vi "设备配置&联机测试.vi"(8 "error in (no error)":errorcluster caption="错误输入（无错误）") -> (0 "error out":errorcluster caption="错误输出")   [LabVIEW 2016]
uses:
  <vilib>/Utility/miscctls.llb/LVPointTypeDef.ctl
  <vilib>/ptbypt/NI_PtbyPt.lvlib
panel:
  in  "关闭":bool
  in  "联机测试":bool
  in  "选项卡控件":T1(tab)
  in  "设备列表":T2(array[cluster])
  out "波特率":u16(ring) items=["300", "600", "1200", "2400", "4800", "9600", "19200", "38400", "115200"]
  out "串口号":u16(ring) items=["COM8", "COM7", "COM6", "COM5", "COM4", "COM3", "COM2", "COM1"]
  out "就绪":bool
  in  "联机":bool
  out "航向":string
  out "速率":string
  out "经度":string
  out "纬度":string
  out "UTC时间":string
  out "UTC日期":string
  out "定位信息":string
  out "串口号 2":u16(ring) items=["COM8", "COM7", "COM6", "COM5", "COM4", "COM3", "COM2", "COM1"]
  out "就绪 2":bool
  in  "联机 2":bool caption="联机"
  in  "选项卡控件 2":T3(tab)
  in  "Turn All OFF":bool
  in  "Apply All":bool
  in  "Read Alarm Sensors":bool
  in  "Control Devices":cluster{"Name":string, "开关":bool, "状态":bool}[](array[cluster])
  in  "报警":cluster{"Name":string, " Status":bool}[](array[cluster])
  in  "Read All Sensor Values":bool
  out "T(cool)℃":string
  out "P（eq)mv":string
  out "R(Gas)mv":string
  out "F(Flow)ml/min":string
  in  "Port2":bool
  in  "Port4":bool
  in  "Port6":bool
  in  "Port8":bool
  out "串口号 4":u16(ring) items=["COM8", "COM7", "COM6", "COM5", "COM4", "COM3", "COM2", "COM1"]
  out "就绪 4":bool
  in  "联机 4":bool caption="联机"
  in  "Go":bool
  in  "Port1":bool
  in  "Port3":bool
  in  "Port5":bool
  in  "Port7":bool
  out "平均次数":dbl
  out "波特率  2":u16(ring) items=["300", "600", "1200", "2400", "4800", "9600", "19200", "38400", "115200"]
  out "串口号 3":u16(ring) items=["COM8", "COM7", "COM6", "COM5", "COM4", "COM3", "COM2", "COM1"]
  out "就绪 3":bool
  in  "联机 3":bool caption="联机"
  out "读数间隔（ms）":dbl
  out "Temperature":string
  out "Conductivity":string
  out "Salinity":string
  out "波特率":u16(ring) items=["300", "600", "1200", "2400", "4800", "9600", "19200", "38400", "115200"]
  out "串口号":u16(ring) items=["COM8", "COM7", "COM6", "COM5", "COM4", "COM3", "COM2", "COM1"]
  out "就绪 5":bool
  in  "联机 5":bool caption="联机"
  out "读数间隔 （ms）":dbl
  out "平均次数":dbl caption="数值"
  out "13CO2":string
  out "13CO2（dry）":string
  out "12CO2":string
  out "12CO2(dry）":string
  out "H2O":string
  out "Delta2Min":string
  out "Delta5Min":string
  out "波特率  3":u16(ring) items=["300", "600", "1200", "2400", "4800", "9600", "19200", "38400", "115200"]
  out "串口号":u16(ring) items=["COM8", "COM7", "COM6", "COM5", "COM4", "COM3", "COM2", "COM1"]
  out "就绪 6":bool
  in  "联机 6":bool caption="联机"
  out "读数间隔":dbl
  out "平均次数":dbl caption="数值"
  out "波特率":u16(ring) items=["300", "600", "1200", "2400", "4800", "9600", "19200", "38400", "115200"]
  out "串口号":u16(ring) items=["COM8", "COM7", "COM6", "COM5", "COM4", "COM3", "COM2", "COM1"]
  out "就绪 7":bool
  in  "联机 7":bool caption="联机"
  out "读数间隔":dbl
  out "平均次数":dbl caption="数值"
  in  "联机 8":bool caption="联机"
  out "就绪 8":bool
  out "串口号":u16(ring) items=["COM8", "COM7", "COM6", "COM5", "COM4", "COM3", "COM2", "COM1"]
  out "波特率":u16(ring) items=["300", "600", "1200", "2400", "4800", "9600", "19200", "38400", "115200"]
  out "时间":string
  out "d15NA":string
  out "d15N":string
  out "N2O":string
  out "d18O":string
  out "H2O":string
  out "d15NB":string
  out "温度摄氏度":string
  out "气压Torr":string
  out "超时us":string
  # "当前GPS信息"
  # "设置"
  # "设置"
  # "Read Temperature/Pressure sensors"
  # "逆转到1、3、5、7"
  # "设置"
  # "设置"
  # "就绪4"
  # "设置"
  # "DATA"
  # "设置"
  # "设置"
  # "设置"
  # "DATA"
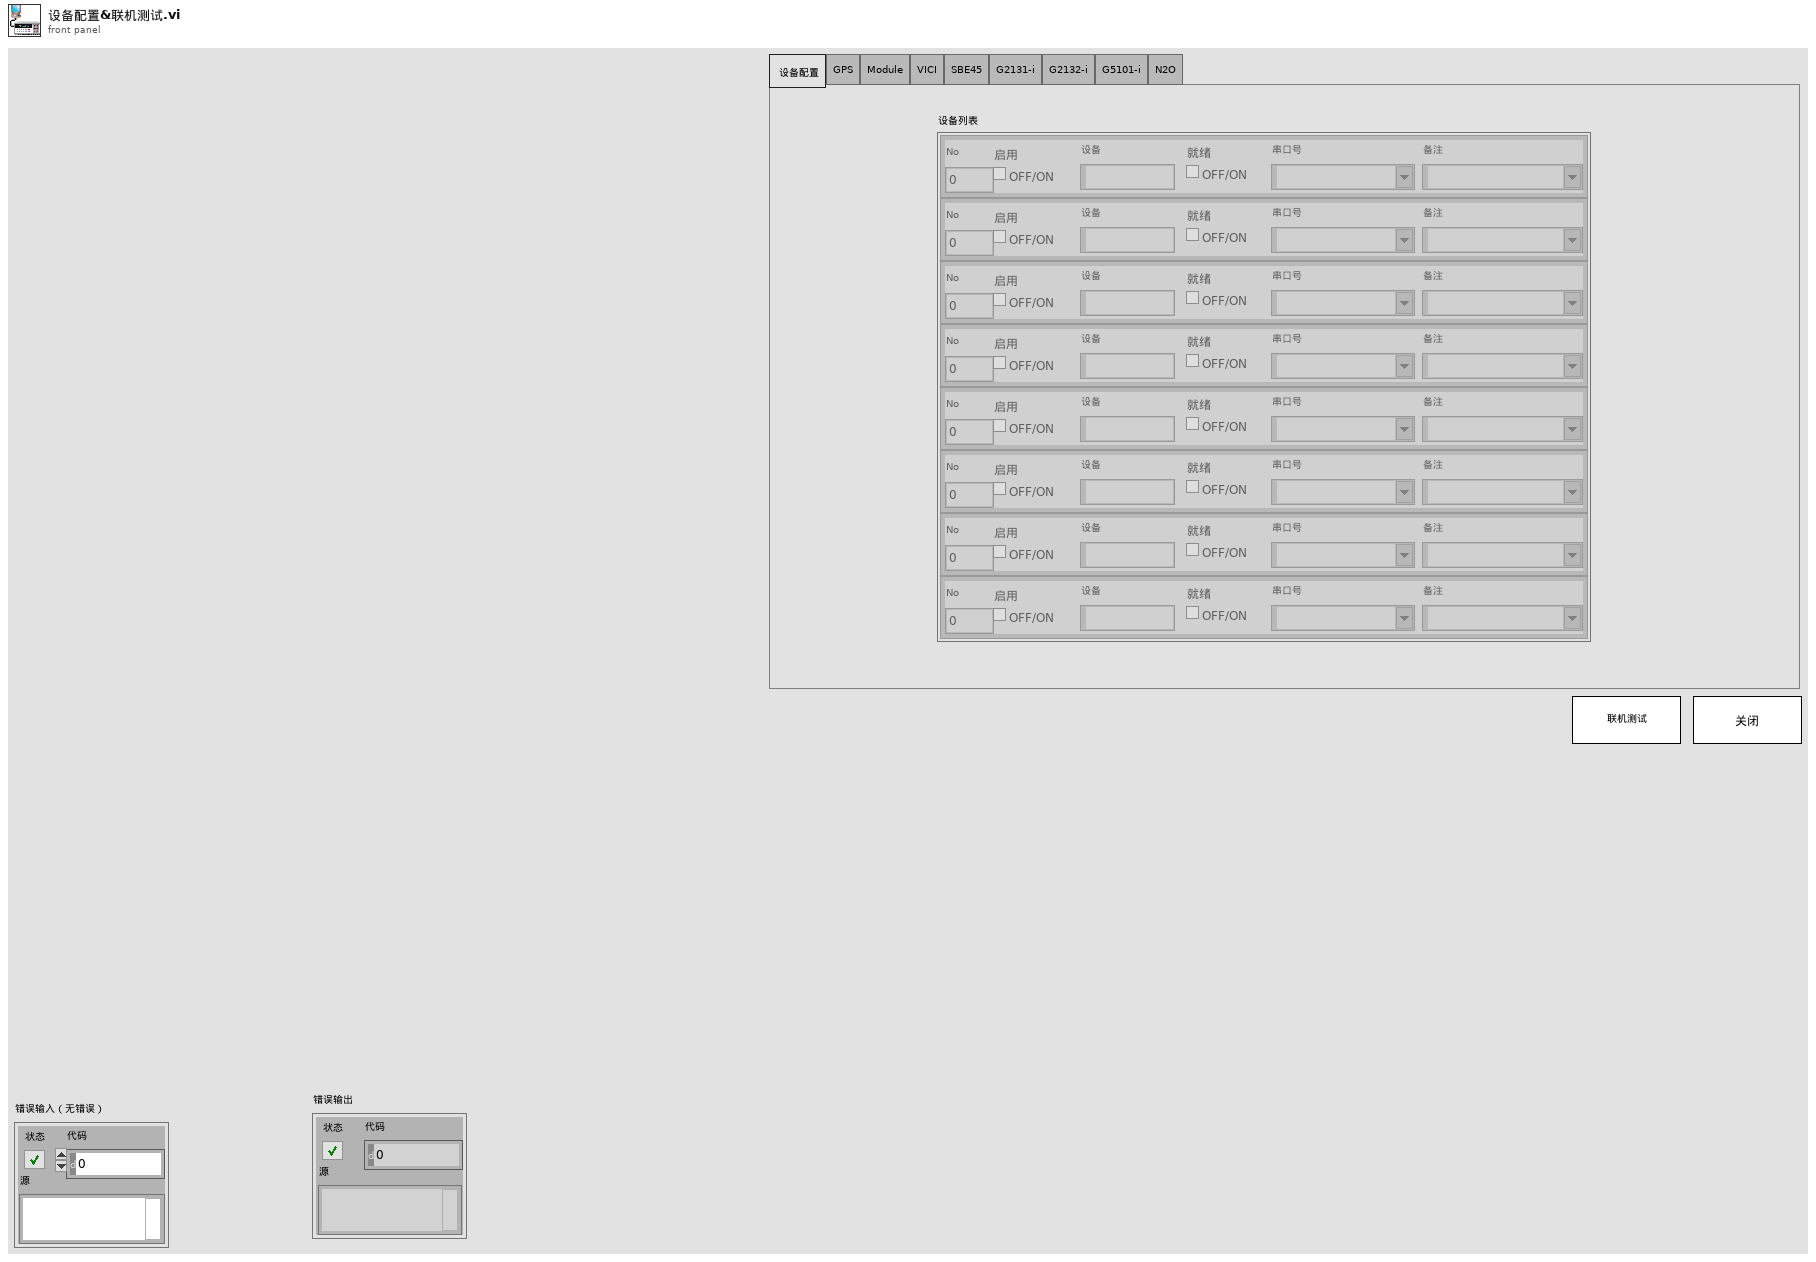
[diagram p1: front panel]
types:
  T1 = enum32{" 设备配置", "GPS", "Module", "VICI", "SBE45", "G2131-i", "G2132-i", "G5101-i", "N2O"}
  T2 = cluster{"No":dbl, "启用":bool, "设备":string, "就绪 ":bool, "串口号":string, "备注":string}[]
  T3 = enum32{"Control Devices&Other Sensors", "T|P|R|F Sensors"}
  T4 = typedef "LVPointTypeDef.ctl" = cluster{"Horizontal":i16, "Vertical":i16}
  T5 = cluster{"No":dbl, "启用":bool, "设备":string, "就绪 ":bool, "串口号":string, "备注":string}
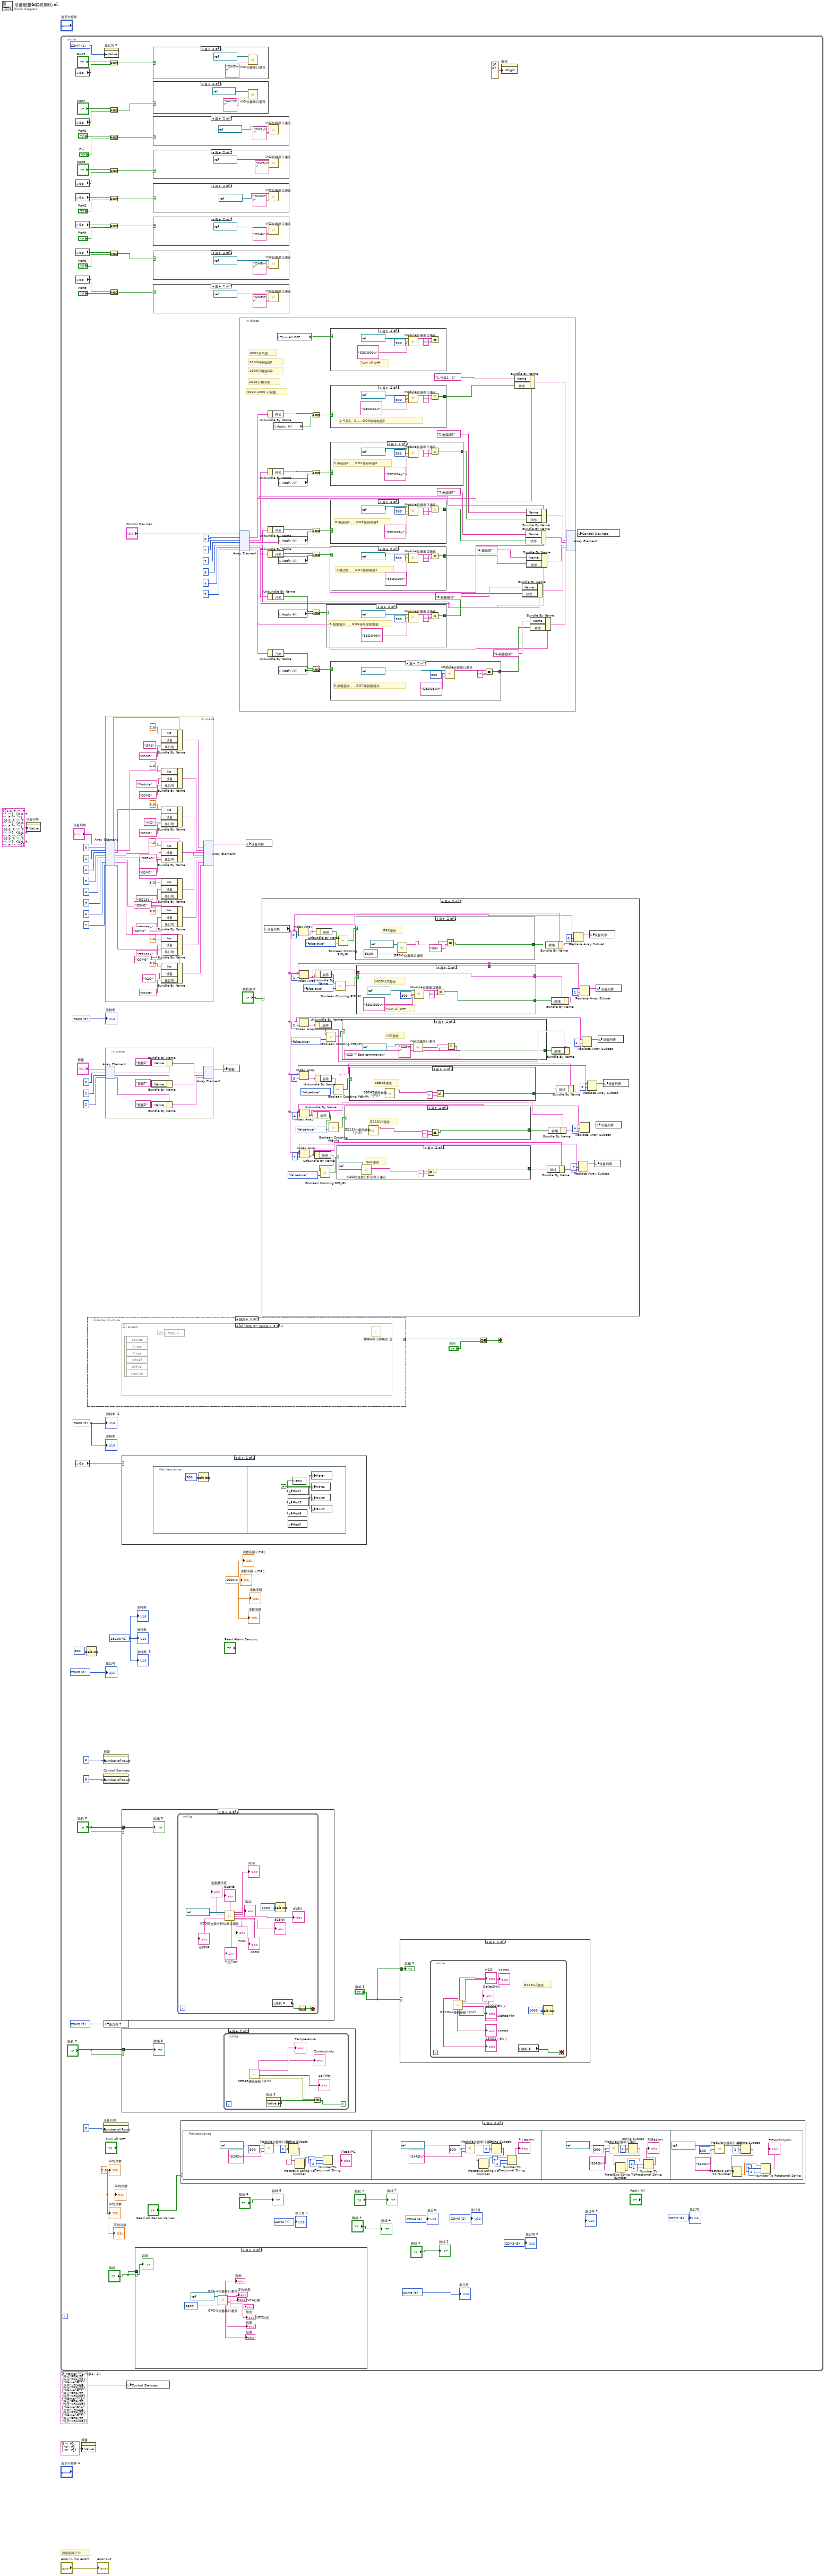
[diagram p0: block diagram]
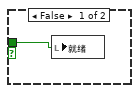
[diagram p9: hidden frame]
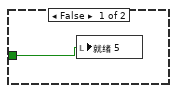
[diagram p10: hidden frame]
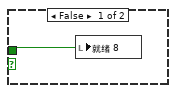
[diagram p11: hidden frame]
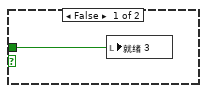
[diagram p17: hidden frame]
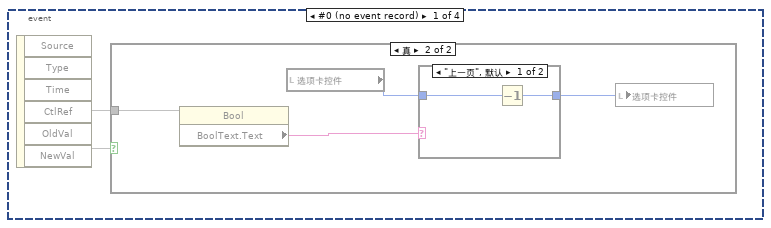
[diagram p18: hidden frame]
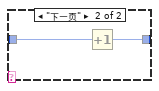
[diagram p20: hidden frame]
diagram:
  # "调用各种子VI"
  n1 = property on="设备列表" class="Arr (严格)"("Value"=T2 [{"No"=1.0, "启用"=FALSE, "设备"="", "就绪 "=FALSE, "串口号"="", "备注"=""}, {"No"=0.0, "启用"=FALSE, "设备"="", "就绪 "=FALSE, "串口号"="", "备注"=""}, {"No"=0.0, "启用"=FALSE, "设备"="", "就绪 "=FALSE, "串口号"="", "备注"=""}, {"No"=0.0, "启用"=FALSE, "设备"="", "就绪 "=FALSE, "串口号"="", "备注"=""}, {"No"=0.0, "启用"=FALSE, "设备"="", "就绪 "=FALSE, "串口号"="", "备注"=""}, {"No"=0.0, "启用"=FALSE, "设备"="", "就绪 "=FALSE, "串口号"="", "备注"=""}, {"No"=0.0, "启用"=FALSE, "设备"="", "就绪 "=FALSE, "串口号"="", "备注"=""}, {"No"=0.0, "启用"=FALSE, "设备"="", "就绪 "=FALSE, "串口号"="", "备注"=""}] ("设备列表")) -> ()  [unwired: 2 in, 2 out]
  n2 = while {
    stop <- w48 stop-if-true
    w12 = u16 5 items=["COM8", "COM7", "COM6", "COM5", "COM4", "COM3", "COM2", "COM1"] ("串口号 2")
    w14 = 1.0 ("平均次数")
    w13 = 1000.0 ("读数间隔 2")
    w18 = u16 2 items=["COM8", "COM7", "COM6", "COM5", "COM4", "COM3", "COM2", "COM1"] ("串口号 7")
    w19 = u16 4 items=["COM8", "COM7", "COM6", "COM5", "COM4", "COM3", "COM2", "COM1"] ("串口号 6")
    w20 = u16 6 items=["COM8", "COM7", "COM6", "COM5", "COM4", "COM3", "COM2", "COM1"] ("串口号 5")
    w21 = u16 7 items=["COM8", "COM7", "COM6", "COM5", "COM4", "COM3", "COM2", "COM1"] ("串口号 4")
    w23 = u16 5 items=["300", "600", "1200", "2400", "4800", "9600", "19200", "38400", "115200"] ("波特率  5")
    w24 = u16 0 items=["COM8", "COM7", "COM6", "COM5", "COM4", "COM3", "COM2", "COM1"] ("串口号 8")
    w26 = u16 5 items=["300", "600", "1200", "2400", "4800", "9600", "19200", "38400", "115200"] ("波特率")
    w27 = u16 6 items=["300", "600", "1200", "2400", "4800", "9600", "19200", "38400", "115200"] ("波特率  4")
    w15 = u16 3 items=["COM8", "COM7", "COM6", "COM5", "COM4", "COM3", "COM2", "COM1"] ("串口号")
    w42 = u16 5 items=["COM8", "COM7", "COM6", "COM5", "COM4", "COM3", "COM2", "COM1"] ("串口号 2")
    w43 = u16 1 items=["COM8", "COM7", "COM6", "COM5", "COM4", "COM3", "COM2", "COM1"] ("串口号 3")
    n3 = local read "Go"() -> (w52:bool)
    n4 = local read "Go"() -> (w51:bool)
    n5 = local read "Go"() -> (w53:bool)
    n6 = local read "Go"() -> (w41:bool)
    n7 = local read "Go"() -> (w38:bool)
    n8 = local read "Go"() -> (w35:bool)
    n9 = local read "Go"() -> (w32:bool)
    n10 = local read "Go"() -> (w29:bool)
    n11 = Wait (ms)(milliseconds to wait=u32 300 ("等待时间（毫秒）")) -> ()  [unwired: 1 out]
    n12 = disable-structure shown="禁用" {
      disable-tunnel: [w226 _] -> w49
      frame Disabled {
        n13 = event shown="[2] \"联机 2\": 值改变" {
          selector: _ -> [_ _ _ _]
          dyn-events: _ -> [_ _ _ _]
          timeout: _ -> [_ _ _ _]
          tunnel: [_ _ _ TRUE] -> w226
          event #0 (no event record) {
            n14 = event-data() -> ("CtlRef"=w228, "NewVal"=w227)  [unwired: 1 in, 4 out]
            n15 = case shown="真" w227 {
              tunnel: w228 -> [_ w232]
              frame False {
              }
              frame True {
                n16 = property class="Bool"(reference=w232) -> ("BoolText.Text"=w231:string)  [unwired: 1 in, 2 out]
                n17 = local read "选项卡控件"() -> (w230:T1)
                n18 = case shown="\"上一页\", 默认" w231 {
                  tunnel: w230 -> [w234 w236]
                  tunnel: [w233 w235] -> w229
                  frame "上一页", Default {
                    n19 = Decrement(x=w234) -> (x-1=w233:T1)
                  }
                  frame "下一页" {
                    n20 = Increment(x=w236) -> (x+1=w235:T1)
                  }
                }
                n21 = local write "选项卡控件"(w229) -> ()
              }
            }
          }
          event #1 (no event record) {
            n22 = event-data() -> ("CtlRef"=w238, "OldVal"=w237)  [unwired: 1 in, 4 out]
            n23 = case shown="真" w237 {
              tunnel: w238 -> [_ w242]
              frame False {
              }
              frame True {
                n24 = property class="Bool (严格)"(reference=w242) -> ("BoolText.Text"=w241:string)  [unwired: 1 in, 2 out]
                n25 = local read "选项卡控件"() -> (w240:T1)
                n26 = case shown="\"下一页\", 默认" w241 {
                  tunnel: w240 -> [w244 w246]
                  tunnel: [w243 w245] -> w239
                  frame "下一页", Default {
                    n27 = Increment(x=w244) -> (x+1=w243:T1)
                  }
                  frame "上一页" {
                    n28 = Decrement(x=w246) -> (x-1=w245:T1)
                  }
                }
                n29 = local write "选项卡控件"(w239) -> ()
              }
            }
          }
          event "联机 2": Value Change {
            n30 = event-data() -> ()  [unwired: 1 in, 6 out]
            n31 = local write "联机 2"(FALSE) -> ()
            n32 = call "模块1串口初始化.vi"() -> ()  [unwired: 12 in]
          }
          event "关闭": Value Change {
            n33 = event-data() -> ()  [unwired: 1 in, 6 out]
          }
        }
      }
      frame Enabled {
      }
    }
    n34 = property on="报警" class="Arr (严格)"("Number of Rows"=u32 3 ("行数")) -> ()  [unwired: 2 in, 2 out]
    n35 = property on="Control Devices" class="Arr (严格)"("Number of Rows"=u32 6 ("行数")) -> ()  [unwired: 2 in, 2 out]
    n36 = property on="设备列表" class="Arr (严格)"("Number of Rows"=u32 8 ("行数")) -> ()  [unwired: 2 in, 2 out]
    n37 = local write "串口号 2"(w42) -> ()
    n38 = property on="串口号 3" class="Ring (严格)"("Value"=w43) -> ()  [unwired: 2 in, 2 out]
    n39 = in-place {
      n40 = in-place-array #1("设备列表", 0, 1, 2 ("数值"), 3, 4, 5, 6, 7) -> (w424:T5, w423:T5, w422:T5, w416:T5, w410:T5, w409:T5, w405:T5, w398:T5)
      n41 = Bundle By Name(cluster=w424, "No"=1.0 ("数值"), "设备"="GPS" ("字符串"), "串口号"="COM5") -> (w430:T5)
      n42 = Bundle By Name(cluster=w423, "No"=2.0, "设备"="Module", "串口号"="COM3") -> (w425:T5)
      n43 = Bundle By Name(cluster=w422, "No"=3.0, "设备"="VICI", "串口号"="COM1") -> (w421:T5)
      n44 = Bundle By Name(cluster=w416, "No"=4.0, "设备"="SBE45", "串口号"="COM7") -> (w415:T5)
      n45 = Bundle By Name(cluster=w410, "No"=5.0, "设备"="G2131-i", "串口号"="COM2") -> (w408:T5)
      n46 = Bundle By Name(cluster=w409, "No"=6.0, "设备"="G2132-i", "串口号"="COM4") -> (w407:T5)
      n47 = Bundle By Name(cluster=w405, "No"=7.0, "设备"="G5101-i", "串口号"="COM6") -> (w404:T5)
      n48 = Bundle By Name(cluster=w398, "No"=8.0, "设备"="N2O", "串口号"="COM8") -> (w397:T5)
      n49 = in-place-array #1(w430, w425, w421, w415, w408, w407, w404, w397) -> (w77:T2)  [unwired: 8 out]
    }
    n50 = in-place {
      n51 = in-place-array #2("报警", 0, 1, 2) -> (w305:cluster{"Name":string, " Status":bool}, w302:cluster{"Name":string, " Status":bool}, w299:cluster{"Name":string, " Status":bool})
      n52 = Bundle By Name(cluster=w305, "Name"="报警1") -> (w304:cluster{"Name":string, " Status":bool})
      n53 = Bundle By Name(cluster=w302, "Name"="报警2") -> (w301:cluster{"Name":string, " Status":bool})
      n54 = Bundle By Name(cluster=w299, "Name"="报警3") -> (w300:cluster{"Name":string, " Status":bool})
      n55 = in-place-array #2(w304, w301, w300) -> (w62:cluster{"Name":string, " Status":bool}[])  [unwired: 3 out]
    }
    n56 = And(x="Port5", y=w52) -> (x .and. y?=w55:bool)
    n57 = And(x="Port7", y=w51) -> (x .and. y?=w54:bool)
    n58 = And(x="Port1", y="Go") -> (x .and. y?=w57:bool)
    n59 = And(x="Port3", y=w53) -> (x .and. y?=w56:bool)
    n60 = And(x=w41, y="Port2") -> (x .and. y?=w39:bool)
    n61 = And(x=w38, y="Port4") -> (x .and. y?=w36:bool)
    n62 = And(x=w35, y="Port6") -> (x .and. y?=w33:bool)
    n63 = And(x=w32, y="Port8") -> (x .and. y?=w30:bool)
    n64 = case shown="真" w29 {
      frame False {
      }
      frame True {
        n65 = flat-sequence {
          frame #0 {
            n66 = Wait (ms)(milliseconds to wait=u32 500 ("等待时间（毫秒）")) -> ()  [unwired: 1 out]
          }
          frame #1 {
            w209 = FALSE
            n67 = local write "Port1"(w209) -> ()
            n68 = local write "Port3"(w209) -> ()
            n69 = local write "Port5"(w209) -> ()
            n70 = local write "Port7"(w209) -> ()
            n71 = local write "Go"(w209) -> ()
            n72 = local write "Port4"(w209) -> ()
            n73 = local write "Port6"(w209) -> ()
            n74 = local write "Port8"(w209) -> ()
            n75 = local write "Port2"(w209) -> ()
          }
        }
      }
    }
    n76 = case shown="真" "联机 8" {
      tunnel: "联机 8" -> [w192 w193]
      frame False {
        n77 = local write "就绪 8"(w192) -> ()
      }
      frame True {
        n78 = while {
          stop <- w203 stop-if-true
          n79 = call "N2O同位素分析仪串口通讯.vi"("VISA resource name"=refnum<visa-resource-name> "COM8") -> ("温度摄氏度"=→"温度摄氏度":string, "d15NB"=→"d15NB":string, "时间"=→"时间":string, "N2O"=→"N2O":string, "d15N"=→"d15N":string, "d18O"=→"d18O":string, "超时us"=→"超时us":string, "气压Torr"=→"气压Torr":string, "H2O"=→"H2O":string, "d15NA"=→"d15NA":string)  [unwired: 5 in]
          n80 = local read "联机 8"() -> (w204:bool)
          n81 = Wait (ms)(milliseconds to wait=u32 1000 ("等待时间（毫秒）")) -> ()  [unwired: 1 out]
          n82 = Not(x=w204) -> (.not. x?=w203:bool)
        }
        "就绪 8" <- w193
      }
    }
    n83 = case shown="真" "联机 3" {
      tunnel: "联机 3" -> [w218 w219]
      frame False {
        n84 = local write "就绪 3"(w218) -> ()
      }
      frame True {
        n85 = while {
          stop <- w221 continue-if-true
          n86 = call "SBE45通讯参数 (子VI).vi"() -> ("错误输出"=w222:errorcluster, "Salinity"=→"Salinity":string, "Conductivity"=→"Conductivity":string, "Temperature"=→"Temperature":string)  [unwired: 8 in]
          n87 = property on="联机 3" class="Bool (严格)"() -> ("Value"=w220:bool)  [unwired: 2 in, 2 out]
          n88 = Or(x=w222, y=w220) -> (x .or. y?=w221:bool)
        }
        "就绪 3" <- w219
      }
    }
    n89 = case shown="真" "联机" {
      selector: "联机" -> [_ w178]
      tunnel: "联机" -> [w168 _]
      frame False {
        n90 = local write "就绪"(w168) -> ()
      }
      frame True {
        n91 = call "GPS-1仪器串口通讯.vi"("VISA resource name"=refnum<visa-resource-name> "COM5", "baud rate (9600)"=u32 9600) -> ()  [unwired: 10 in, 8 out]
        n92 = call "GPS-1仪器串口通讯.vi"("VISA resource name"=refnum<visa-resource-name> "COM5", "baud rate (9600)"=u32 9600) -> ("速率"=→"速率":string, "经度"=→"经度":string, "定位信息"=→"定位信息":string, "UTC日期"=→"UTC日期":string, "航向"=→"航向":string, "UTC时间"=→"UTC时间":string, "纬度"=→"纬度":string)  [unwired: 10 in, 1 out]
        "就绪" <- w178
      }
    }
    n93 = case shown="真" w55 {
      frame False {
      }
      frame True {
        n94 = call "VICI仪器串口通讯.vi"("输入指令"="CW5\n\r", "VISA resource name"=refnum<visa-resource-name> "COM1") -> ()  [unwired: 1 in, 3 out]
      }
    }
    n95 = case shown="真" w54 {
      frame False {
      }
      frame True {
        n96 = call "VICI仪器串口通讯.vi"("输入指令"="CW7\n\r", "VISA resource name"=refnum<visa-resource-name> "COM1") -> ()  [unwired: 1 in, 3 out]
      }
    }
    n97 = case shown="真" w57 {
      frame False {
      }
      frame True {
        n98 = call "VICI仪器串口通讯.vi"("输入指令"="CW1\n\r", "VISA resource name"=refnum<visa-resource-name> "COM1") -> ()  [unwired: 1 in, 3 out]
      }
    }
    n99 = case shown="真" w56 {
      frame False {
      }
      frame True {
        n100 = call "VICI仪器串口通讯.vi"("输入指令"="CW3\n\r", "VISA resource name"=refnum<visa-resource-name> "COM1") -> ()  [unwired: 1 in, 3 out]
      }
    }
    n101 = case shown="真" w39 {
      frame False {
      }
      frame True {
        n102 = call "VICI仪器串口通讯.vi"("输入指令"="CW2\n\r", "VISA resource name"=refnum<visa-resource-name> "COM1") -> ()  [unwired: 1 in, 3 out]
      }
    }
    n103 = case shown="真" w36 {
      frame False {
      }
      frame True {
        n104 = call "VICI仪器串口通讯.vi"("输入指令"="CW4\r", "VISA resource name"=refnum<visa-resource-name> "COM1") -> ()  [unwired: 1 in, 3 out]
      }
    }
    n105 = case shown="真" w33 {
      frame False {
      }
      frame True {
        n106 = call "VICI仪器串口通讯.vi"("输入指令"="CW6\n\r", "VISA resource name"=refnum<visa-resource-name> "COM1") -> ()  [unwired: 1 in, 3 out]
      }
    }
    n107 = case shown="真" w30 {
      frame False {
      }
      frame True {
        n108 = call "VICI仪器串口通讯.vi"("输入指令"="CW8\n\r", "VISA resource name"=refnum<visa-resource-name> "COM1") -> ()  [unwired: 1 in, 3 out]
      }
    }
    n109 = case shown="真" "Read All Sensor Values" {
      frame False {
      }
      frame True {
        n110 = flat-sequence {
          frame #0 {
            n111 = call "Module仪器串口通讯.vi"("输入指令"="$2RD\r", "baud rate"=u32 300 ("baud rate (9600)"), "VISA resource name"=refnum<visa-resource-name> "COM3") -> ("子字符串;substring"=w254:string)  [unwired: 2 out]
            n112 = String Subset(string=w254, offset (0)=2 ("偏移量(0)")) -> (substring=w253:string)  [unwired: 1 in]
            n113 = Fract/Exp String To Number(string=w253) -> (number=w252:dbl)  [unwired: 3 in, 1 out]
            n114 = Number To Fractional String(number=w252, width (-)=i16 2 ("宽度(-)"), precision (6)=i16 2 ("精度(6)")) -> (F-format string=→"T(cool)℃":string)  [unwired: 1 in]
          }
          frame #1 {
            n115 = call "Module仪器串口通讯.vi"("输入指令"="$4RD\r", "baud rate"=u32 300 ("baud rate (9600)"), "VISA resource name"=refnum<visa-resource-name> "COM3") -> ("子字符串;substring"=w264:string)  [unwired: 2 out]
            n116 = String Subset(string=w264, offset (0)=2 ("偏移量(0)")) -> (substring=w260:string)  [unwired: 1 in]
            n117 = Fract/Exp String To Number(string=w260) -> (number=w263:dbl)  [unwired: 3 in, 1 out]
            n118 = Number To Fractional String(number=w263, width (-)=i16 2 ("宽度(-)"), precision (6)=i16 2 ("精度(6)")) -> (F-format string=→"P（eq)mv":string)  [unwired: 1 in]
          }
          frame #2 {
            n119 = call "Module仪器串口通讯.vi"("输入指令"="$5RD\r", "baud rate"=u32 300 ("baud rate (9600)"), "VISA resource name"=refnum<visa-resource-name> "COM3") -> ("子字符串;substring"=w274:string)  [unwired: 2 out]
            n120 = String Subset(string=w274, offset (0)=2 ("偏移量(0)")) -> (substring=w270:string)  [unwired: 1 in]
            n121 = Fract/Exp String To Number(string=w270) -> (number=w271:dbl)  [unwired: 3 in, 1 out]
            n122 = Number To Fractional String(number=w271, width (-)=i16 2 ("宽度(-)"), precision (6)=i16 2 ("精度(6)")) -> (F-format string=→"R(Gas)mv":string)  [unwired: 1 in]
          }
          frame #3 {
            n123 = call "Module仪器串口通讯.vi"("输入指令"="$6RD\r", "baud rate"=u32 300 ("baud rate (9600)"), "VISA resource name"=refnum<visa-resource-name> "COM3") -> ("子字符串;substring"=w288:string)  [unwired: 2 out]
            n124 = String Subset(string=w288, offset (0)=2 ("偏移量(0)")) -> (substring=w280:string)  [unwired: 1 in]
            n125 = Fract/Exp String To Number(string=w280) -> (number=w283:dbl)  [unwired: 3 in, 1 out]
            n126 = Number To Fractional String(number=w283, width (-)=i16 2 ("宽度(-)"), precision (6)=i16 2 ("精度(6)")) -> (F-format string=→"F(Flow)ml/min":string)  [unwired: 1 in]
          }
        }
      }
    }
    n127 = local write "报警"(w62) -> ()
    n128 = in-place {
      # "0010 1000 开报警"
      # "1010开蠕动泵"
      # "1000开电磁阀2"
      # "0100开电磁阀1"
      # "0001开气泵"
      n129 = in-place-array #3("Control Devices", 0, 1, 2, 3, 4, 5) -> (w319:cluster{"Name":string, "开关":bool, "状态":bool}, w320:cluster{"Name":string, "开关":bool, "状态":bool}, w321:cluster{"Name":string, "开关":bool, "状态":bool}, w327:cluster{"Name":string, "开关":bool, "状态":bool}, w332:cluster{"Name":string, "开关":bool, "状态":bool}, w331:cluster{"Name":string, "开关":bool, "状态":bool})
      n130 = Unbundle By Name(w319) -> ("开关"=w322:bool)
      n131 = Unbundle By Name(w320) -> ("开关"=w323:bool)
      n132 = Unbundle By Name(w321) -> ("开关"=w326:bool)
      n133 = Unbundle By Name(w327) -> ("开关"=w330:bool)
      n134 = Unbundle By Name(w332) -> ("开关"=w336:bool)
      n135 = Unbundle By Name(w331) -> ("开关"=w333:bool)
      n136 = local read "Apply All"() -> (w306:bool)
      n137 = local read "Turn All OFF"() -> (w318:bool)
      n138 = local read "Apply All"() -> (w324:bool)
      n139 = local read "Apply All"() -> (w325:bool)
      n140 = local read "Apply All"() -> (w329:bool)
      n141 = local read "Apply All"() -> (w335:bool)
      n142 = local read "Apply All"() -> (w310:bool)
      n143 = And(x=w322, y=w306) -> (x .and. y?=w307:bool)
      n144 = And(x=w323, y=w324) -> (x .and. y?=w308:bool)
      n145 = And(x=w326, y=w325) -> (x .and. y?=w309:bool)
      n146 = And(x=w330, y=w329) -> (x .and. y?=w328:bool)
      n147 = And(x=w336, y=w335) -> (x .and. y?=w334:bool)
      n148 = And(x=w333, y=w310) -> (x .and. y?=w317:bool)
      n149 = case shown="真" w334 {
        tunnel: [_ w385] -> w314
        frame False {
        }
        frame True {
          # "5.报警器开，，DO6接外部报警器"
          n150 = call "Module仪器串口通讯.vi"("输入指令"="$3DO40\r", "baud rate"=u32 300 ("baud rate (9600)"), "VISA resource name"=refnum<visa-resource-name> "COM3") -> ("子字符串;substring"=w386:string)  [unwired: 2 out]
          n151 = Equal?(x=w386, y="*") -> (x = y?=w385:bool)
        }
      }
      n152 = case shown="真" w318 {
        frame False {
        }
        frame True {
          # "Turn All OFF"
          n153 = call "Module仪器串口通讯.vi"("输入指令"="$3DO00\r", "baud rate"=u32 300 ("baud rate (9600)"), "VISA resource name"=refnum<visa-resource-name> "COM3") -> ("子字符串;substring"=w349:string)  [unwired: 2 out]
          n154 = Equal?(x=w349, y="*") -> ()  [unwired: 1 out]
        }
      }
      n155 = case shown="真" w307 {
        tunnel: [_ w354] -> w316
        frame False {
        }
        frame True {
          # "1.气泵1、2,,,,,,DO0接继电器0"
          n156 = call "Module仪器串口通讯.vi"("输入指令"="$3DO01\r", "baud rate"=u32 300 ("baud rate (9600)"), "VISA resource name"=refnum<visa-resource-name> "COM3") -> ("子字符串;substring"=w355:string)  [unwired: 2 out]
          n157 = Equal?(x=w355, y="*") -> (x = y?=w354:bool)
        }
      }
      n158 = case shown="真" w308 {
        tunnel: [FALSE w361] -> w311
        frame False {
        }
        frame True {
          # "2.电磁阀1，，DO2接继电器2"
          n159 = call "Module仪器串口通讯.vi"("输入指令"="$3DO04\r", "baud rate"=u32 300 ("baud rate (9600)"), "VISA resource name"=refnum<visa-resource-name> "COM3") -> ("子字符串;substring"=w362:string)  [unwired: 2 out]
          n160 = Equal?(x=w362, y="*") -> (x = y?=w361:bool)
        }
      }
      n161 = case shown="真" w309 {
        tunnel: [_ w367] -> w312
        frame False {
        }
        frame True {
          # "3.电磁阀2，，DO3接继电器3"
          n162 = call "Module仪器串口通讯.vi"("输入指令"="$3DO08\r", "baud rate"=u32 300 ("baud rate (9600)"), "VISA resource name"=refnum<visa-resource-name> "COM3") -> ("子字符串;substring"=w368:string)  [unwired: 2 out]
          n163 = Equal?(x=w368, y="*") -> (x = y?=w367:bool)
        }
      }
      n164 = case shown="真" w328 {
        tunnel: [_ w373] -> w313
        frame False {
        }
        frame True {
          # "4.蠕动泵，，DO4接继电器4"
          n165 = call "Module仪器串口通讯.vi"("输入指令"="$3DO10\r", "baud rate"=u32 300 ("baud rate (9600)"), "VISA resource name"=refnum<visa-resource-name> "COM3") -> ("子字符串;substring"=w374:string)  [unwired: 2 out]
          n166 = Equal?(x=w374, y="*") -> (x = y?=w373:bool)
        }
      }
      n167 = case shown="真" w317 {
        tunnel: [_ w379] -> w315
        frame False {
        }
        frame True {
          # "6.报警器关，，DO7接报警器关"
          n168 = call "Module仪器串口通讯.vi"("输入指令"="$3DO80\r", "baud rate"=u32 300 ("baud rate (9600)"), "VISA resource name"=refnum<visa-resource-name> "COM3") -> ("子字符串;substring"=w380:string)  [unwired: 2 out]
          n169 = Equal?(x=w380, y="*") -> (x = y?=w379:bool)
        }
      }
      n170 = Bundle By Name(cluster=w319, "Name"="1.气泵1、2" ("字符串"), "状态"=w316) -> (w348:cluster{"Name":string, "开关":bool, "状态":bool})
      n171 = Bundle By Name(cluster=w332, "Name"="5.报警器开" ("字符串"), "状态"=w314) -> (w338:cluster{"Name":string, "开关":bool, "状态":bool})
      n172 = Bundle By Name(cluster=w321, "Name"="3.电磁阀2" ("字符串"), "状态"=w312) -> (w340:cluster{"Name":string, "开关":bool, "状态":bool})
      n173 = Bundle By Name(cluster=w320, "Name"="2.电磁阀1" ("字符串"), "状态"=w311) -> (w341:cluster{"Name":string, "开关":bool, "状态":bool})
      n174 = Bundle By Name(cluster=w327, "Name"="4.蠕动泵" ("字符串"), "状态"=w313) -> (w339:cluster{"Name":string, "开关":bool, "状态":bool})
      n175 = Bundle By Name(cluster=w331, "Name"="6.报警器关" ("字符串"), "状态"=w315) -> (w337:cluster{"Name":string, "开关":bool, "状态":bool})
      n176 = in-place-array #3(w348, w341, w340, w339, w338, w337) -> (w72:cluster{"Name":string, "开关":bool, "状态":bool}[])  [unwired: 6 out]
    }
    n177 = local write "设备列表"(w77) -> ()
    n178 = case shown="真" "联机测试" {
      frame False {
      }
      frame True {
        n179 = local read "设备列表"() -> (w106:T2)
        n180 = Index Array(array=w106, index=0 ("索引")) -> (element=w125:T5)
        n181 = Index Array(array=w106, index=2 ("索引")) -> (element=w120:T5)
        n182 = Index Array(array=w106, index=3 ("索引")) -> (element=w117:T5)
        n183 = Index Array(array=w106, index=1 ("索引")) -> (element=w139:T5)
        n184 = Index Array(array=w106, index=4 ("索引")) -> (element=w110:T5)
        n185 = Index Array(array=w106, index=7 ("索引")) -> (element=w107:T5)
        n186 = Unbundle By Name(w110) -> ("启用"=w85:bool)
        n187 = Unbundle By Name(w107) -> ("启用"=w87:bool)
        n188 = Unbundle By Name(w120) -> ("启用"=w94:bool)
        n189 = Unbundle By Name(w139) -> ("启用"=w102:bool)
        n190 = Unbundle By Name(w117) -> ("启用"=w91:bool)
        n191 = Unbundle By Name(w125) -> ("启用"=w98:bool)
        n192 = call <vilib>:"Boolean Crossing PtByPt.vi"("direction"=enum16{"either", "false-true", "true-false"}."false-true", "input"=w87) -> ("crossing"=w88:bool)  [unwired: 1 in]
        n193 = call <vilib>:"Boolean Crossing PtByPt.vi"("direction"=enum16{"either", "false-true", "true-false"}."false-true", "input"=w94) -> ("crossing"=w95:bool)  [unwired: 1 in]
        n194 = call <vilib>:"Boolean Crossing PtByPt.vi"("direction"=enum16{"either", "false-true", "true-false"}."false-true", "input"=w85) -> ("crossing"=w86:bool)  [unwired: 1 in]
        n195 = call <vilib>:"Boolean Crossing PtByPt.vi"("direction"=enum16{"either", "false-true", "true-false"}."false-true", "input"=w91) -> ("crossing"=w92:bool)  [unwired: 1 in]
        n196 = call <vilib>:"Boolean Crossing PtByPt.vi"("direction"=enum16{"either", "false-true", "true-false"}."false-true", "input"=w102) -> ("crossing"=w101:bool)  [unwired: 1 in]
        n197 = case shown="真" w88 {
          tunnel: [_ w141] -> w105
          frame False {
          }
          frame True {
            # "N2O通信"
            n198 = call "N2O同位素分析仪串口通讯.vi"("VISA resource name"=refnum<visa-resource-name> "COM8") -> ("时间"=w143:string)  [unwired: 5 in, 9 out]
            n199 = Not Equal?(x=w143, y="") -> (x != y?=w141:bool)
          }
        }
        n200 = call <vilib>:"Boolean Crossing PtByPt.vi"("direction"=enum16{"either", "false-true", "true-false"}."false-true", "input"=w98) -> ("crossing"=w97:bool)  [unwired: 1 in]
        n201 = case shown="真" w95 {
          tunnel: [_ w151] -> w119
          frame False {
          }
          frame True {
            # "VICI通信"
            n202 = call "VICI仪器串口通讯.vi"("输入指令"="CC3\n\r", "VISA resource name"=refnum<visa-resource-name> "COM1") -> ("read buffer"=w153:string)  [unwired: 1 in, 2 out]
            n203 = Equal?(x=w153, y="CC3 = Bad command\r") -> (x = y?=w151:bool)
          }
        }
        n204 = case shown="真" w86 {
          tunnel: [_ w145] -> w109
          frame False {
          }
          frame True {
            # "G2131-i通信"
            n205 = call "G2131-i通讯参数 (子VI).vi"() -> ("12CO2"=w146:string)  [unwired: 5 in, 6 out]
            n206 = Not Equal?(x=w146, y="") -> (x != y?=w145:bool)
          }
        }
        n207 = case shown="真" w92 {
          tunnel: [_ w148] -> w116
          frame False {
          }
          frame True {
            # "SBE45通信"
            n208 = call "SBE45通讯参数 (子VI).vi"() -> ("Temperature"=w149:string)  [unwired: 8 in, 3 out]
            n209 = Not Equal?(x=w149, y="") -> (x != y?=w148:bool)
          }
        }
        n210 = case shown="真" w97 {
          tunnel: [_ w163] -> w124
          frame False {
          }
          frame True {
            # "GPS通信"
            n211 = call "GPS-1仪器串口通讯.vi"("VISA resource name"=refnum<visa-resource-name> "COM5", "baud rate (9600)"=u32 9600) -> ("定位信息"=w165:string)  [unwired: 10 in, 7 out]
            n212 = Not Equal?(x=w165, y="N/A") -> (x != y?=w163:bool)
          }
        }
        n213 = case shown="真" w101 {
          tunnel: w139 -> [_ w157]
          tunnel: w106 -> [_ _]
          tunnel: [_ w157] -> w130
          tunnel: [_ w156] -> w129
          frame False {
          }
          frame True {
            # "Turn All OFF"
            # "MODULE通信"
            n214 = call "Module仪器串口通讯.vi"("输入指令"="$3DO00\r", "baud rate"=u32 300 ("baud rate (9600)"), "VISA resource name"=refnum<visa-resource-name> "COM3") -> ("子字符串;substring"=w162:string)  [unwired: 2 out]
            n215 = Equal?(x=w162, y="*") -> (x = y?=w156:bool)
          }
        }
        n216 = Bundle By Name(cluster=w125, "就绪"=w124) -> (w128:T5)
        n217 = Bundle By Name(cluster=w107, "就绪"=w105) -> (w104:T5)
        n218 = Bundle By Name(cluster=w110, "就绪"=w109) -> (w111:T5)
        n219 = Bundle By Name(cluster=w130, "就绪"=w129) -> (w133:T5)
        n220 = Bundle By Name(cluster=w120, "就绪"=w119) -> (w123:T5)
        n221 = Bundle By Name(cluster=w117, "就绪"=w116) -> (w115:T5)
        n222 = Replace Array Subset(array=w106, new element=w128, index=0 ("索引")) -> (w127:T2)
        n223 = Replace Array Subset(array=w106, new element=w104, index=7 ("索引")) -> (w103:T2)
        n224 = Replace Array Subset(array=w106, new element=w133, index=1 ("索引")) -> (w132:T2)
        n225 = Replace Array Subset(array=w106, new element=w111, index=4 ("索引")) -> (w113:T2)
        n226 = Replace Array Subset(array=w106, new element=w123, index=2 ("索引")) -> (w122:T2)
        n227 = Replace Array Subset(array=w106, new element=w115, index=3 ("索引")) -> (w114:T2)
        n228 = local write "设备列表"(w127) -> ()
        n229 = local write "设备列表"(w103) -> ()
        n230 = local write "设备列表"(w132) -> ()
        n231 = local write "设备列表"(w113) -> ()
        n232 = local write "设备列表"(w122) -> ()
        n233 = local write "设备列表"(w114) -> ()
      }
    }
    n234 = case shown="真" "联机 5" {
      tunnel: "联机 5" -> [w181 w182]
      frame False {
        n235 = local write "就绪 5"(w181) -> ()
      }
      frame True {
        n236 = while {
          stop <- w183 stop-if-true
          # "G2131-i通信"
          n237 = call "G2131-i通讯参数 (子VI).vi"() -> ("12CO2(dry）"=→"12CO2(dry）":string, "Delta2Min"=→"Delta2Min":string, "12CO2"=→"12CO2":string, "Delta5Min"=→"Delta5Min":string, "H2O"=→"H2O":string, "13CO2"=→"13CO2":string, "13CO2（dry）"=→"13CO2（dry）":string)  [unwired: 5 in]
          n238 = local read "联机 5"() -> (w183:bool)
          n239 = Wait (ms)(milliseconds to wait=u32 1000 ("等待时间（毫秒）")) -> ()  [unwired: 1 out]
        }
        "就绪 5" <- w182
      }
    }
    n240 = Or(x=w49, y="关闭") -> (x .or. y?=w48:bool)
    n241 = property on="窗格" class="Pane"("Origin"=T4 {"Horizontal"=0, "Vertical"=0} ("原点")) -> ()  [unwired: 2 in, 2 out]
    n242 = local write "Control Devices"(w72) -> ()
    "串口号" <- w15
    "波特率" <- w26
    "就绪 2" <- "联机 2"
    "平均次数" <- w14
    "读数间隔" <- w13
    "就绪 6" <- "联机 6"
    "就绪 7" <- "联机 7"
    "串口号 2" <- w12
    "波特率  2" <- w26
    "就绪 4" <- "联机 4"
    "串口号 4" <- w21
    "平均次数" <- w14
    "串口号" <- w20
    "波特率" <- w27
    "平均次数" <- w14
    "串口号" <- w19
    "波特率  3" <- w27
    "串口号" <- w18
    "波特率" <- w27
    "读数间隔 （ms）" <- w13
    "读数间隔" <- w13
    "读数间隔（ms）" <- w13
    "平均次数" <- w14
    "串口号" <- w24
    "波特率" <- w23
  }
  n243 = property on="报警" class="Arr (严格)"("Value"=cluster{"Name":string, " Status":bool}[] [{"Name"="", " Status"=FALSE}, {"Name"="0", " Status"=FALSE}, {"Name"="0", " Status"=FALSE}] ("数组")) -> ()  [unwired: 2 in, 2 out]
  n244 = local write "Control Devices"(cluster{"Name":string, "开关":bool, "布尔":bool}[] [{"Name"="1.气泵1、2", "开关"=FALSE, "布尔"=FALSE}, {"Name"="1", "开关"=FALSE, "布尔"=FALSE}, {"Name"="2", "开关"=FALSE, "布尔"=FALSE}, {"Name"="3", "开关"=FALSE, "布尔"=FALSE}, {"Name"="4", "开关"=FALSE, "布尔"=FALSE}, {"Name"="5", "开关"=FALSE, "布尔"=FALSE}] ("Control Devices")) -> ()
  "error out" <- "error in (no error)"
